vi "Check File & Folder .vi"(8 "error in (no error)":errorcluster) -> (0 "error out":errorcluster, 2 "Path 2":T1, 3 "Config Path":path)   [LabVIEW 2023]
uses:
  Controls/all path.ctl
panel:
  out "calbration date":timestamp
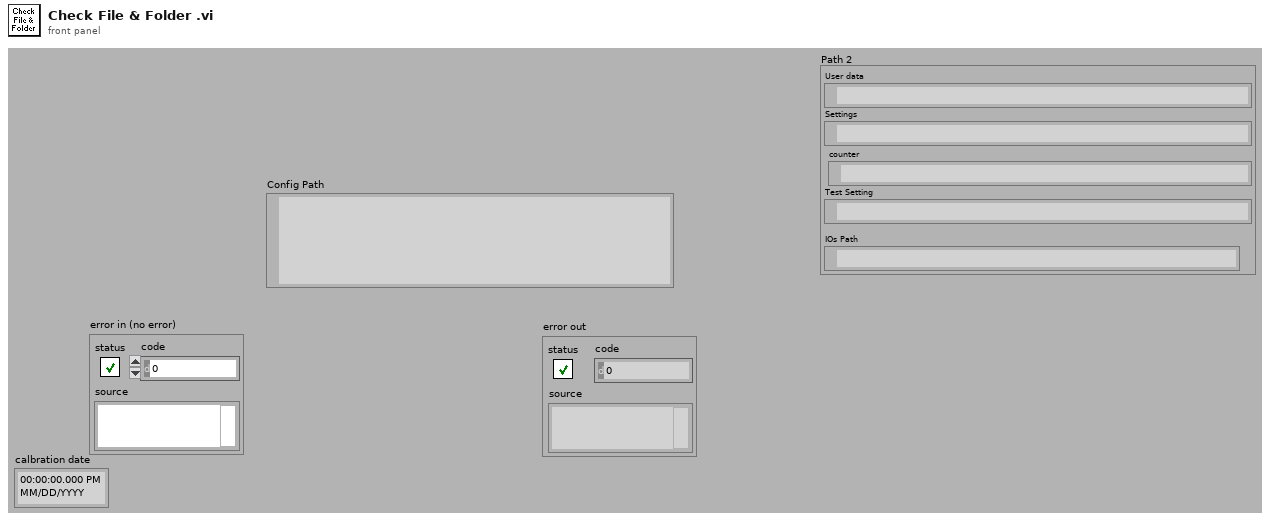
[diagram p1: front panel]
types:
  T1 = typedef "all path.ctl" = cluster{"User data":path, "Settings":path, "counter":path, "Test Setting":path, "IOs Path":path}
  T2 = cluster{"User data":path, "Settings":path, "Calib":path, "Test Setting":path, "IOs config":path}
  T3 = enum16{"open", "replace", "create", "open or create", "replace or create", "replace or create with confirmation"}
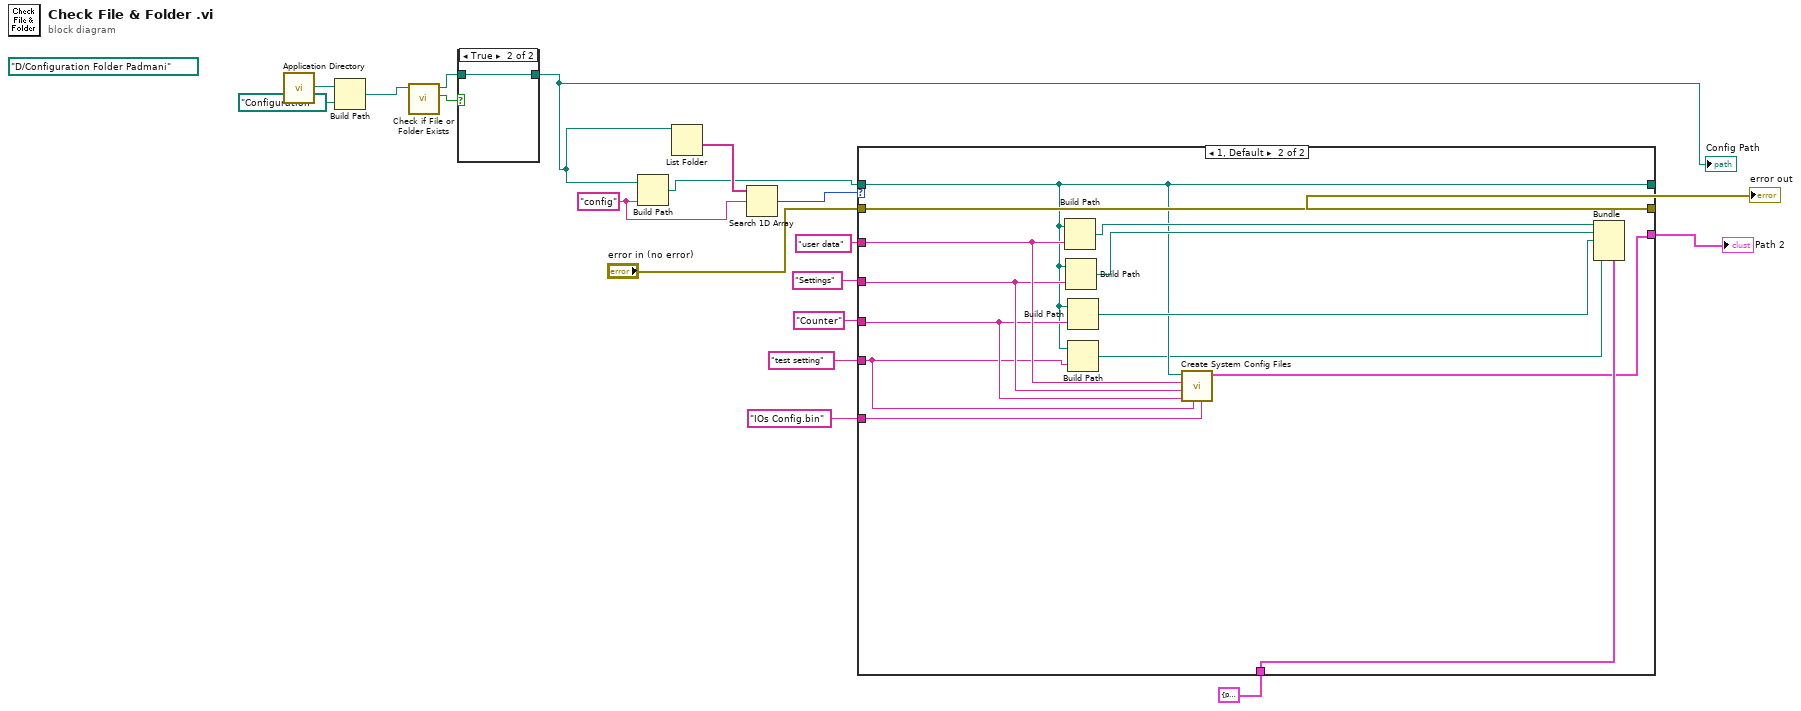
[diagram p0: block diagram]
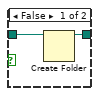
[diagram p2: hidden frame]
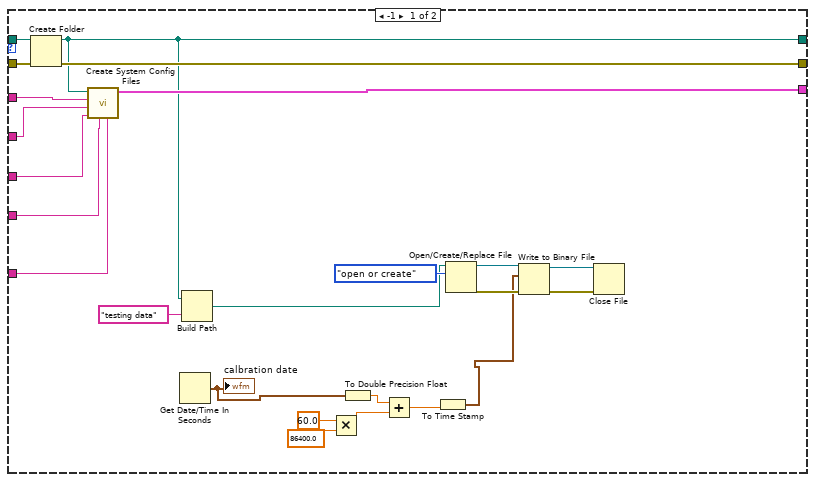
[diagram p3: hidden frame]
diagram:
  (unwired) path "D:/Configuration Folder Padmani" ("path")
  w17 = "config"
  n1 = call <vilib>:"Application Directory.vi"() -> ("Application Directory"=w3:path)
  n2 = Build Path(base path=w3, name or relative path=path "Configuration") -> (appended path=w1:path)
  n3 = call <vilib>:"Check if File or Folder Exists.vi"("path"=w1) -> ("file or folder exists?"=w6:bool, "dup path"=w5:path)  [unwired: 8 in, 1 out]
  n4 = case shown="True" w6 {
    tunnel: w5 -> [w21 w22]
    tunnel: [w20 w22] -> w4
    frame False {
      n5 = Create Folder(path (use dialog)=w21) -> (created path=w20:path)  [unwired: 2 in, 2 out]
    }
    frame True {
    }
  }
  "Config Path" <- w4
  n6 = Build Path(base path=w4, name or relative path=w17) -> (appended path=w14:path)
  n7 = List Folder(path=w4) -> (folder names=w18:string[])  [unwired: 1 in, 5 out]
  n8 = Search 1D Array(1D array=w18, element=w17) -> (index of element=w16:i32)  [unwired: 1 out]
  n9 = case shown="1, Default" w16 {
    tunnel: w14 -> [w45 w51]
    tunnel: "error in (no error)" -> [w46 w59]
    tunnel: [w31 w51] -> _
    tunnel: [w44 w59] -> w19
    tunnel: [w43 w48] -> w11
    tunnel: "user data" ("User Data") -> [w42 w55]
    tunnel: "Settings" ("Settings") -> [w41 w54]
    tunnel: T2 {"User data"=path "", "Settings"=path "", "Calib"=path "", "Test Setting"=path "", "IOs config"=path ""} ("Path 2") -> [_ w57]
    tunnel: "Counter" ("Settings") -> [w40 w53]
    tunnel: "test setting" ("Test Setting") -> [w39 w50]
    tunnel: "IOs Config.bin" ("Test Setting") -> [w38 w47]
    frame -1 {
      n10 = Create Folder(path (use dialog)=w45, error in=w46) -> (created path=w31:path, error out=w44:errorcluster)  [unwired: 2 out]
      n11 = call "Create System Config Files.vi"("IO's config"=w38, "Test Setting"=w39, "count"=w40, "Settings"=w41, "User Data"=w42, "file path (use dialog)"=w31) -> ("Path 2"=w43:T1)  [unwired: 5 out]
      n12 = Get Date/Time In Seconds() -> (seconds since 1Jan1904=w24:timestamp)
      "calbration date" <- w24
      n13 = Build Path(base path=w31, name or relative path="testing data" ("Test Setting")) -> (appended path=w32:path)
      n14 = Multiply(x=60.0, y=86400.0) -> (x*y=w26:dbl)
      n15 = To Double Precision Float(number=w24) -> (double precision float=w29:dbl)
      n16 = Add(x=w29, y=w26) -> (x+y=w27:dbl)
      n17 = To Time Stamp(1:w27) -> (0:w23:timestamp)
      n18 = Open/Create/Replace File(file path (use dialog)=w32, operation (0:open)=T3."open or create") -> (refnum out=w34:refnum<file>, error out=w35:errorcluster)  [unwired: 4 in, 1 out]
      n19 = Write to Binary File(file (use dialog)=w34, data=w23, error in=w35) -> (refnum out=w36:refnum<file>, error out=w37:errorcluster)  [unwired: 3 in, 1 out]
      n20 = Close File(refnum=w36, error in=w37) -> ()  [unwired: 2 out]
    }
    frame 1, Default {
      n21 = Build Path(base path=w51, name or relative path=w55) -> (appended path=w58:path)
      n22 = Build Path(base path=w51, name or relative path=w54) -> (appended path=w56:path)
      n23 = Build Path(base path=w51, name or relative path=w53) -> (appended path=w52:path)
      n24 = Build Path(base path=w51, name or relative path=w50) -> (appended path=w49:path)
      n25 = call "Create System Config Files.vi"("IO's config"=w47, "Test Setting"=w50, "count"=w53, "Settings"=w54, "User Data"=w55, "file path (use dialog)"=w51) -> ("Path 2"=w48:T1)  [unwired: 5 out]
      n26 = Bundle(cluster=w57, "User data"=w58, "Settings"=w56, "Calib"=w52, "Test Setting"=w49) -> ()  [unwired: 1 in, 1 out]
    }
  }
  "error out" <- w19
  "Path 2" <- w11
